vi "Stop Core.vi"(10 "final error code":i32, 11 "CS++DeviceGUIActor in":refnum<class "CS++DSCTrendViewer.lvclass">) -> (3 "CS++DeviceGUIActor out":refnum<class "CS++DSCTrendViewer.lvclass">)   [LabVIEW 2013, in "CS++DSCTrendViewer.lvlib" / "CS++DSCTrendViewer.lvclass"]
doc: "(<B>Filename</B>: Actor Framework.lvlib:Actor.lvclass:Stop Core.vi)\n\nDefines what the actor does before it stops. Use the <B>final error code</B> input to determine whether the actor shut down in response to an error.\n\nBy default, this method does nothing. A descendant class may override it to define behavior, such as shutting down any processes the actor initiated in its override of the Actor Core method."
uses:
  CS++DSCTrendViewer.lvclass
  CS++GUIActor/CS++GUIActor.lvclass
  CS++BaseActor/CS++BaseActor.lvclass/CS++BaseActor.ctl
  CS++DSCTrendViewer.lvclass/CS++DSCTrendViewer.ctl
  CS++BaseActor/CS++BaseActor.lvclass
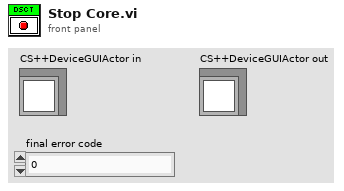
[diagram p1: front panel]
types:
  T1 = enum16{"open", "replace", "create", "open or create", "replace or create", "replace or create with confirmation"}
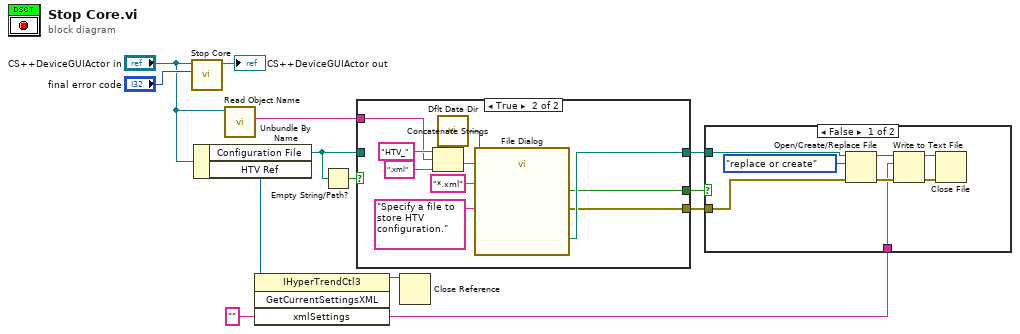
[diagram p0: block diagram]
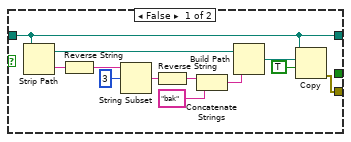
[diagram p3: hidden frame]
diagram:
  n1 = call-parent "Stop Core.vi"("final error code"="final error code", "CS++DeviceGUIActor in"="CS++DeviceGUIActor in") -> ("CS++DeviceGUIActor out"=→"CS++DeviceGUIActor out":refnum<class "CS++DSCTrendViewer.lvclass">)  [unwired: 9 in]
  n2 = Unbundle By Name("CS++DeviceGUIActor in") -> ("Configuration File"=w5:path, "HTV Ref"=w10:refnum<k7>)
  n3 = call "Read Object Name.vi"("CS++BaseActor in"="CS++DeviceGUIActor in") -> ("Object Name"=w1:string)  [unwired: 8 in, 2 out]
  n4 = invoke class="IHyperTrendCtl3" method="GetCurrentSettingsXML"(reference=w10, "xmlSettings"="") -> (reference out=w9:refnum<k7>, "xmlSettings"=w8:string)  [unwired: 2 in, 2 out]
  n5 = Empty String/Path?(string/path=w5) -> (empty?=w6:bool)
  n6 = case shown="True" w6 {
    tunnel: [w15 w34] -> w7
    tunnel: w5 -> [w14 _]
    tunnel: [w14 w35] -> w4
    tunnel: [_ w31] -> w3
    tunnel: w1 -> [_ w27]
    frame False {
      n7 = Strip Path(path=w14) -> (stripped path=w19:path, name=w24:string)
      n8 = Reverse String(1:w24) -> (0:w25:string)
      n9 = String Subset(string=w25, offset (0)=3) -> (substring=w22:string)  [unwired: 1 in]
      n10 = Reverse String(1:w22) -> (0:w21:string)
      n11 = Concatenate Strings(w21, "bak" ("string")) -> (w18:string)
      n12 = Build Path(base path=w19, name or relative path=w18) -> (appended path=w17:path)
      n13 = Copy(9:TRUE ("overwrite (F)"), 10:w17, 11:w14) -> (0:w15:errorcluster)  [unwired: 2 in, 2 out]
    }
    frame True {
      n14 = Concatenate Strings("HTV_" ("default name"), w27, ".xml" ("default name")) -> (w30:string)
      n15 = call <vilib>:"Dflt Data Dir.vi"() -> ("App:Default Data Directory"=w26:path)
      n16 = call "File Dialog"("start path"=w26, "prompt"="Specify a file to store HTV configuration.", "default name"=w30, "pattern (all files)"="*.xml") -> ("selected path"=w35:path, "cancelled"=w31:bool, "error out"=w34:errorcluster)  [unwired: 8 in, 1 out]
    }
  }
  n17 = Close Reference(reference=w9) -> ()  [unwired: 1 in, 1 out]
  n18 = case shown="False" w3 {
    tunnel: w8 -> [w40 _]
    tunnel: w7 -> [w37 _]
    tunnel: w4 -> [w36 _]
    frame False {
      n19 = Open/Create/Replace File(file path (use dialog)=w36, error in=w37, operation (0:open)=T1."replace or create") -> (refnum out=w41:refnum<file>, error out=w42:errorcluster)  [unwired: 3 in, 1 out]
      n20 = Write to Text File(file (use dialog)=w41, text=w40, error in=w42) -> (refnum out=w39:refnum<file>, error out=w38:errorcluster)  [unwired: 1 in, 1 out]
      n21 = Close File(refnum=w39, error in=w38) -> ()  [unwired: 2 out]
    }
    frame True {
    }
  }
